vi "offset_gps_xy_pairs.vi"(1 "offset":dbl, 2 "XY data":cluster{timestamp[], dbl[]}) -> (0 "XY data":cluster{timestamp[], dbl[]})   [LabVIEW 2020]
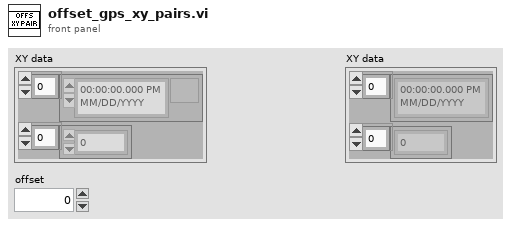
[diagram p1: front panel]
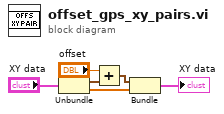
[diagram p0: block diagram]
diagram:
  n1 = Unbundle("XY data") -> (w5:timestamp[], w3:dbl[])
  n2 = Add(x="offset", y=w5) -> (x+y=w4:timestamp[])
  n3 = Bundle(w4, w3) -> (→"XY data":cluster{timestamp[], dbl[]})  [unwired: 1 in]
